vi "N_simu_temp.vi"(9 "Lmini":dbl, 10 "L max":dbl, 11 "N":u32) -> (3 "Array":dbl[](array[numeric]))   [LabVIEW 2020]
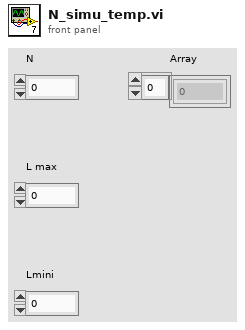
[diagram p1: front panel]
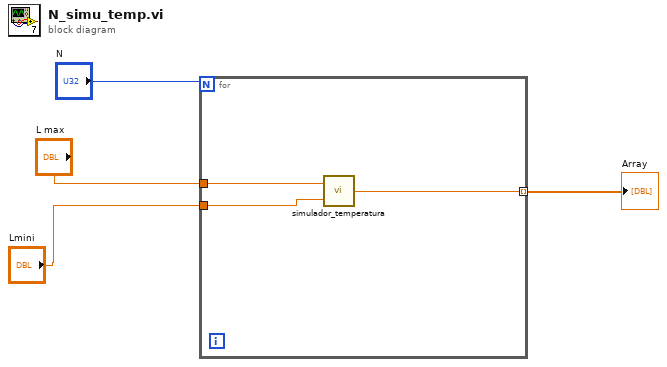
[diagram p0: block diagram]
diagram:
  n1 = for {
    N: "N" -> [_]
    tunnel: "L max" -> [w7]
    tunnel: "Lmini" -> [w6]
    tunnel: [w5] -> w4 mode=indexing
    n2 = call "simulador_temperatura.vi"("L max"=w6, "Lmini"=w7) -> ("Numeric"=w5:dbl)
  }
  "Array" <- w4
